vi "PawnToPiece.vi"() -> (3 "Figure type":T1)   [LabVIEW 2019]
uses:
  #typedef_PieceType.ctl
panel:
  in  "Queen":bool
  in  "Rook":bool
  in  "Bishop":bool
  in  "Knight":bool
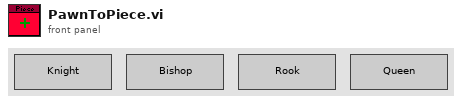
[diagram p1: front panel]
types:
  T1 = typedef "#typedef_PieceType.ctl" = enum16{"None", "Pawn", "Knight", "Bishop", "Rook", "Queen", "King"}
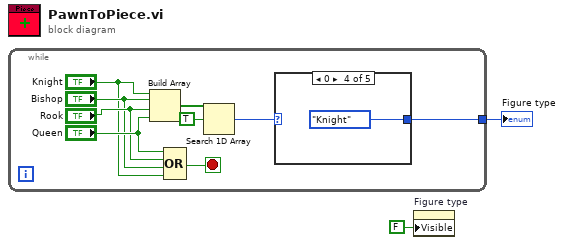
[diagram p0: block diagram]
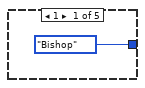
[diagram p2: hidden frame]
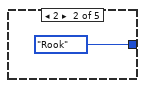
[diagram p3: hidden frame]
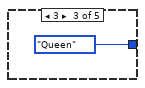
[diagram p4: hidden frame]
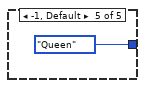
[diagram p5: hidden frame]
diagram:
  n1 = while {
    tunnel: [w3] -> w2
    stop <- w4 stop-if-true
    n2 = Build Array("Knight", "Bishop", "Rook", "Queen") -> (w11:bool[])
    n3 = Compound Arithmetic op=OR("Queen", "Rook", "Bishop", "Knight") -> (w4:bool)
    n4 = Search 1D Array(1D array=w11, element=TRUE) -> (index of element=w9:i32)  [unwired: 1 in]
    n5 = case shown="0" w9 {
      tunnel: [#typedef_PieceType."Bishop" ("Figure type") #typedef_PieceType."Rook" ("Figure type") #typedef_PieceType."Queen" ("Figure type") #typedef_PieceType."Knight" ("Figure type") #typedef_PieceType."Queen" ("Figure type")] -> w3
      frame 1 {
      }
      frame 2 {
      }
      frame 3 {
      }
      frame 0 {
      }
      frame -1, Default {
      }
    }
  }
  "Figure type" <- w2
  n6 = property on="Figure type" class="Enum (strict)"("Visible"=FALSE) -> ()  [unwired: 2 in, 2 out]
